vi "find next action.vi"(10 "desired state":T1, 11 "current state":T1) -> (3 "action":T2)   [LabVIEW 2013, in "main engine.lvlib"]
uses:
  main engine.lvlib
  engine process action.ctl
  <vilib>/NI/Module Execution Interface/Engine Runtime/Execution States.ctl
  <vilib>/NI/Module Execution Interface/Engine Runtime/Engine Runtime Interface.lvclass
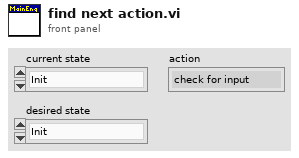
[diagram p1: front panel]
types:
  T1 = typedef "Engine Runtime Interface.lvclass/Execution States.ctl" = enum16{"Init", "Pre-Operational", "Safe-Operational", "Operational", "Stopped"}
  T2 = typedef "main engine.lvlib/engine process action.ctl" = enum16{"check for input", "load configuration", "unload configuration", "set safe outputs", "return to pre", "pre-run", "timed loop", "quit"}
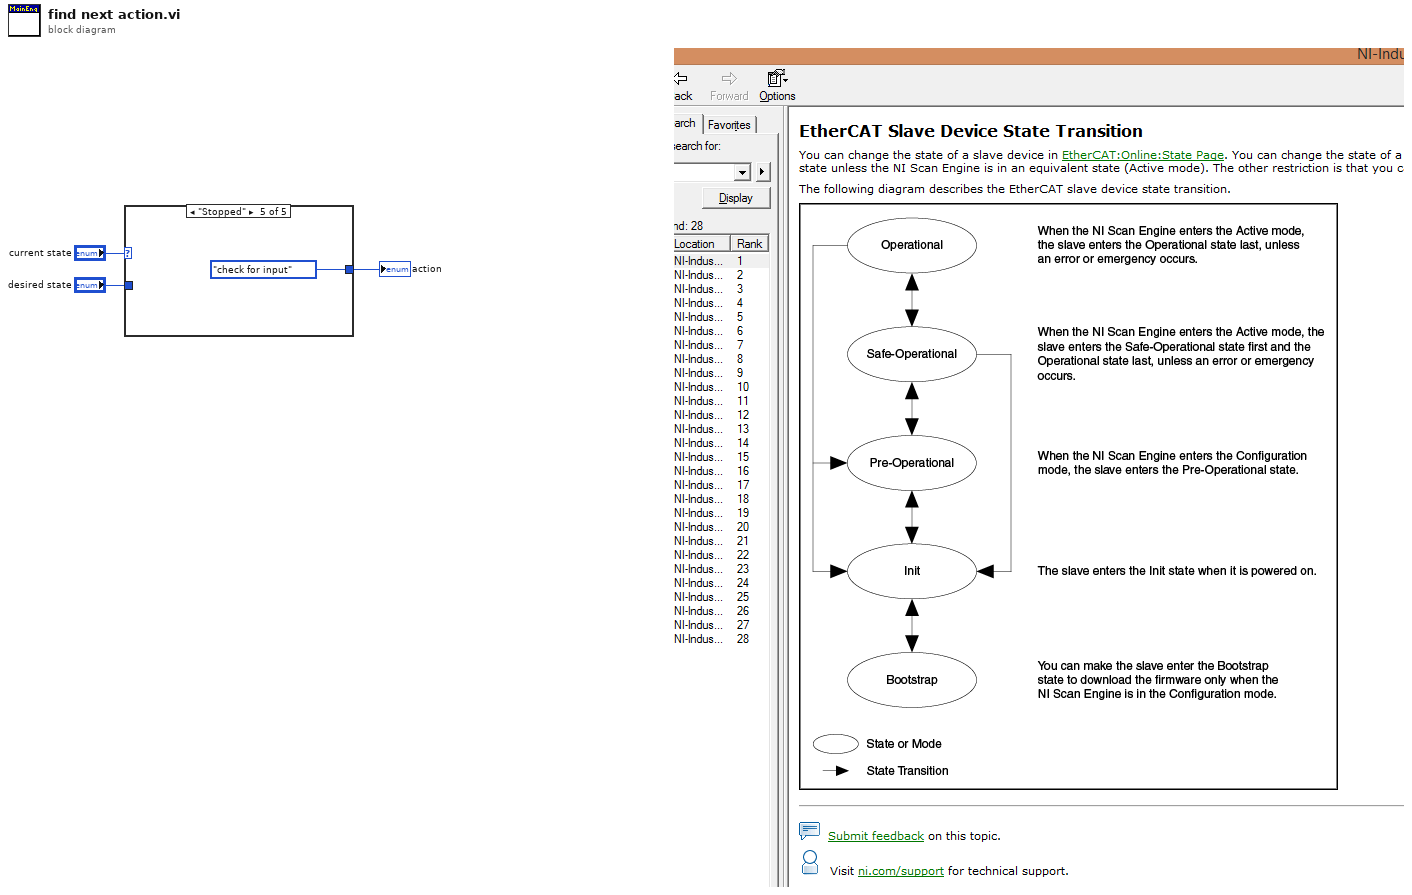
[diagram p0: block diagram]
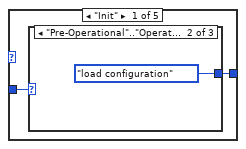
[diagram p2: hidden frame]
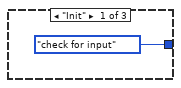
[diagram p3: hidden frame]
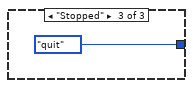
[diagram p4: hidden frame]
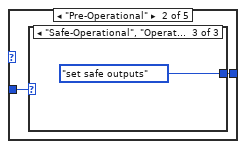
[diagram p5: hidden frame]
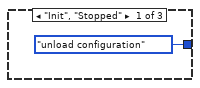
[diagram p6: hidden frame]
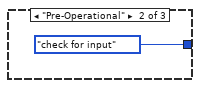
[diagram p7: hidden frame]
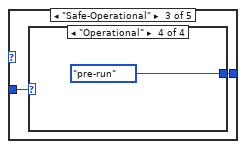
[diagram p8: hidden frame]
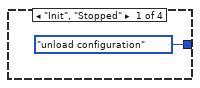
[diagram p9: hidden frame]
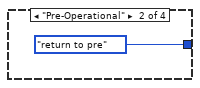
[diagram p10: hidden frame]
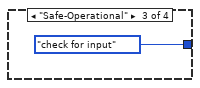
[diagram p11: hidden frame]
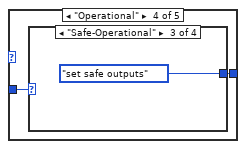
[diagram p12: hidden frame]
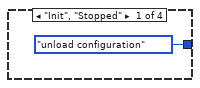
[diagram p13: hidden frame]
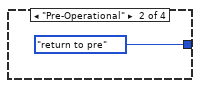
[diagram p14: hidden frame]
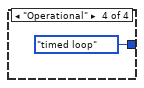
[diagram p15: hidden frame]
diagram:
  n1 = case shown="\"Stopped\"" "current state" {
    tunnel: "desired state" -> [w5 w10 w15 w21 _]
    tunnel: [w4 w9 w14 w20 engine_process_action."check for input"] -> w1
    frame "Init" {
      n2 = case shown="\"Pre-Operational\"..\"Operational\"" w5 {
        tunnel: [engine_process_action."check for input" engine_process_action."load configuration" engine_process_action."quit"] -> w4
        frame "Init" {
        }
        frame "Pre-Operational".."Operational" {
        }
        frame "Stopped" {
        }
      }
    }
    frame "Pre-Operational" {
      n3 = case shown="\"Safe-Operational\", \"Operational\"" w10 {
        tunnel: [engine_process_action."unload configuration" engine_process_action."check for input" engine_process_action."set safe outputs"] -> w9
        frame "Init", "Stopped" {
        }
        frame "Pre-Operational" {
        }
        frame "Safe-Operational", "Operational" {
        }
      }
    }
    frame "Safe-Operational" {
      n4 = case shown="\"Operational\"" w15 {
        tunnel: [engine_process_action."unload configuration" engine_process_action."return to pre" engine_process_action."check for input" engine_process_action."pre-run"] -> w14
        frame "Init", "Stopped" {
        }
        frame "Pre-Operational" {
        }
        frame "Safe-Operational" {
        }
        frame "Operational" {
        }
      }
    }
    frame "Operational" {
      n5 = case shown="\"Safe-Operational\"" w21 {
        tunnel: [engine_process_action."unload configuration" engine_process_action."return to pre" engine_process_action."set safe outputs" engine_process_action."timed loop"] -> w20
        frame "Init", "Stopped" {
        }
        frame "Pre-Operational" {
        }
        frame "Safe-Operational" {
        }
        frame "Operational" {
        }
      }
    }
    frame "Stopped" {
    }
  }
  "action" <- w1
